vi "discharge for capacitor.vi"(6 "c":dbl, 7 "t":dbl, 9 "R":dbl, 10 "Vo":dbl, 11 "E":dbl) -> (3 "discharge for \ncapacitor":dbl)   [LabVIEW 2018]
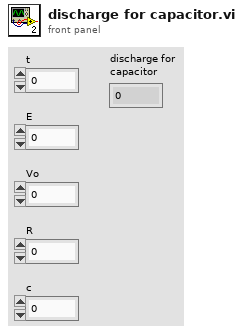
[diagram p1: front panel]
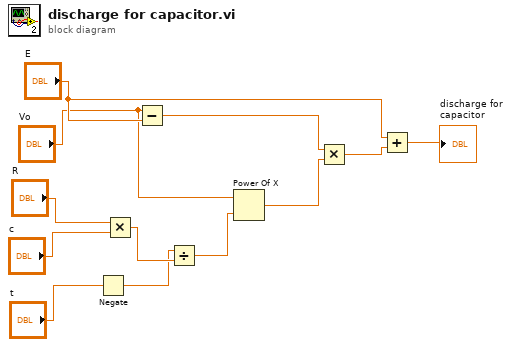
[diagram p0: block diagram]
diagram:
  n1 = Negate(x="t") -> (-x=w4:dbl)
  n2 = Multiply(x="R", y="c") -> (x*y=w5:dbl)
  n3 = Subtract(x="Vo", y="E") -> (x-y=w9:dbl)
  n4 = Divide(x=w4, y=w5) -> (x/y=w6:dbl)
  n5 = Power Of X(1:w6, 2:"Vo") -> (0:w8:dbl)
  n6 = Multiply(x=w9, y=w8) -> (x*y=w10:dbl)
  n7 = Add(x="E", y=w10) -> (x+y=→"discharge for \ncapacitor":dbl)
